vi "Rx UDP Parameter Conversion.vi"(10 "CommPort Payload":T2(array[cluster]) {"Parameters"."encoding" items=["BNR", "BCD", "Discrete"]}, 11 "RxUDPBlockReadInPortArray":T3[](array[typedef]) {"UDP Handle Out" format="%.0x"; "UDP Handle" format="%.0x"}) -> (3 "Values":dbl[](array[numeric]))   [LabVIEW 2024, in "AIM ARINC 664 Engine.lvlib" / "Implementation.lvlib" / "Rx UDP Execution Unit.lvclass"]
uses:
  Rx UDP Execution Unit.lvclass
  <instrlib>/AIM GmbH/_AIM 664/bsp/Controls/ReceiveUDPBlockRead.ctl
  Shared/Encoding (Arinc664).ctl
  Rx UDP Execution Unit.lvclass/Rx UDP Execution Unit.ctl
  <instrlib>/AIM GmbH/_AIM 664/AIM664LV.lvlib
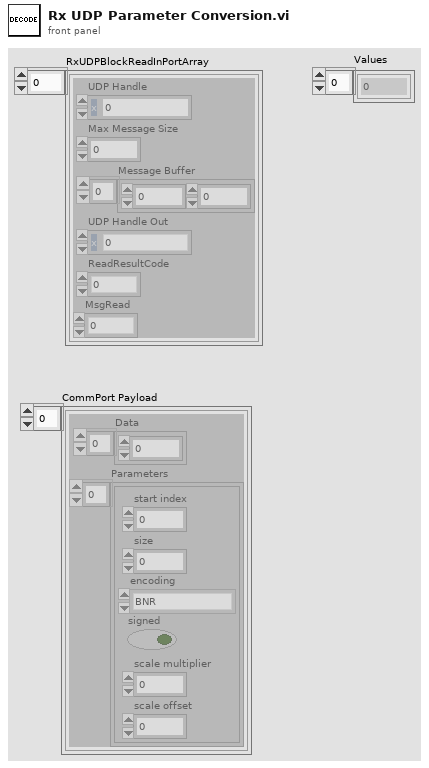
[diagram p1: front panel]
types:
  T1 = typedef "Encoding (Arinc664).ctl" = u16
  T2 = cluster{"Data":u8[], "Parameters":cluster{"start index":i32, "size":i32, "encoding":T1, "signed":bool, "scale multiplier":dbl, "scale offset":dbl}[]}[]
  T3 = typedef "AIM664LV.lvlib/ReceiveUDPBlockRead.ctl" = cluster{"UDP Handle":u32, "Max Message Size":u32, "Message Buffer":u8[], "UDP Handle Out":u32, "ReadResultCode":i32, "MsgRead":u32}
  T4 = cluster{"start index":i32, "size":i32, "encoding":T1, "signed":bool, "scale multiplier":dbl, "scale offset":dbl}[]
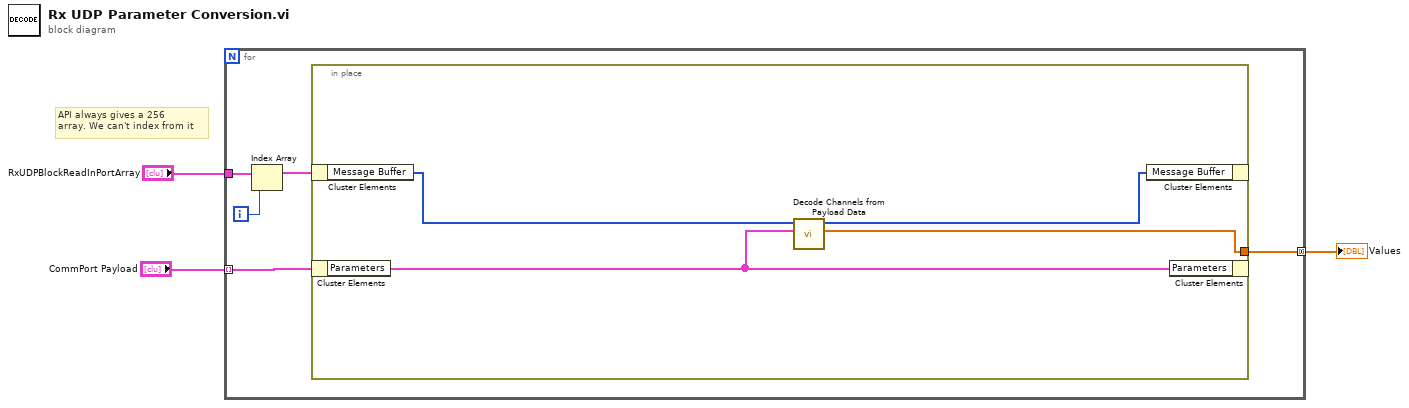
[diagram p0: block diagram]
diagram:
  # "API always gives a 256\narray. We can't index from it"
  n1 = for {
    tunnel: "CommPort Payload" -> [w8] mode=indexing
    tunnel: "RxUDPBlockReadInPortArray" -> [w7]
    tunnel: [w6] -> w1 mode=concatenating
    i -> [w4]
    n2 = Index Array(array=w7, index=w4) -> (element=w5:T3)
    n3 = in-place {
      in-place-border: [w9] -> w6
      n4 = in-place-cluster #1(w5) -> ("Message Buffer"=w12:u8[])
      n5 = in-place-cluster #2(w8) -> ("Parameters"=w10:T4)
      n6 = call "Decode Channels from Payload Data.vi"("Parameters"=w10, "Message Buffer in"=w12) -> ("Channels"=w9:dbl[], "Message Buffer out"=w11:u8[])  [unwired: 8 in]
      n7 = in-place-cluster #1("Message Buffer"=w11) -> ()  [unwired: 1 out]
      n8 = in-place-cluster #2("Parameters"=w10) -> ()  [unwired: 1 out]
    }
  }
  "Values" <- w1
